vi "1_2_UnifiedCameraCalibration.vi"(5 "um/pix conversion method":T6=1 items=["Strip Centers", "Signal Fit, Left to Right", "Projection + Signal Fit"], 7 "Sharpness assessment method":T5=enum."Mean( Laplacian Convolution )", 8 "error in (no error)":errorcluster, 9 "Strip Pitch (microns)":dbl=74.5 format="%#_13g", 10 "Naming Convention":string="*.png", 11 "Images Directory":path) -> (0 "error out":errorcluster, 3 "Camera calibration results":T3 {"Working distance to stave [mm]" format="%#_13g"})   [LabVIEW 2016]
uses:
  Utils/Controls/All_Enums/Enum_TypeDef_ImageSharpnessAnalysisMethod.ctl
  Utils/Controls/All_Enums/Enum_TypeDef_CameraCalibrationResults.ctl
  Utils/Controls/All_Enums/Ring_TypeDef_PixUmConversionMethod.ctl
  Utils/Controls/All_Enums/Enum_TypeDef_ParabolaFitType.ctl
  <vilib>/Utility/file.llb/Read Delimited Spreadsheet (DBL).vi
panel:
  out "IndexNearOptimal":i32
  out "Array 3":dbl[](array[numeric])
  out "Array 2":dbl[](array[numeric])
  out "Array":dbl[](array[numeric])
  out "Images":T1[](array[plugin-control])
  out "Processing Image #":i32
  in  "Tab Control":T2(tab)
  in  "Name of coordinate file":string="XYZcaptured.csv"
  out "Sharpness vs Height":T4(graph)
  out "Uncertainty on height [mm]":dbl
  out "Optimized height [mm]":dbl
  out "Conversion vs Height":cluster{"all rows":dbl[], dbl[]}[](graph)
  out "Conversion [um/pix]":dbl
  out "Uncertainty on conversion":dbl
  # "CALIBRATE CAMERA Brandeis University - Brookhaven National Laboratory * ATLAS Phase II Inner Tracker Upgrade\nPrimary Authors: H. Herde (hherde@brandeis.edu), C. Nicoloff (cnicolof@wellesley.edu)"
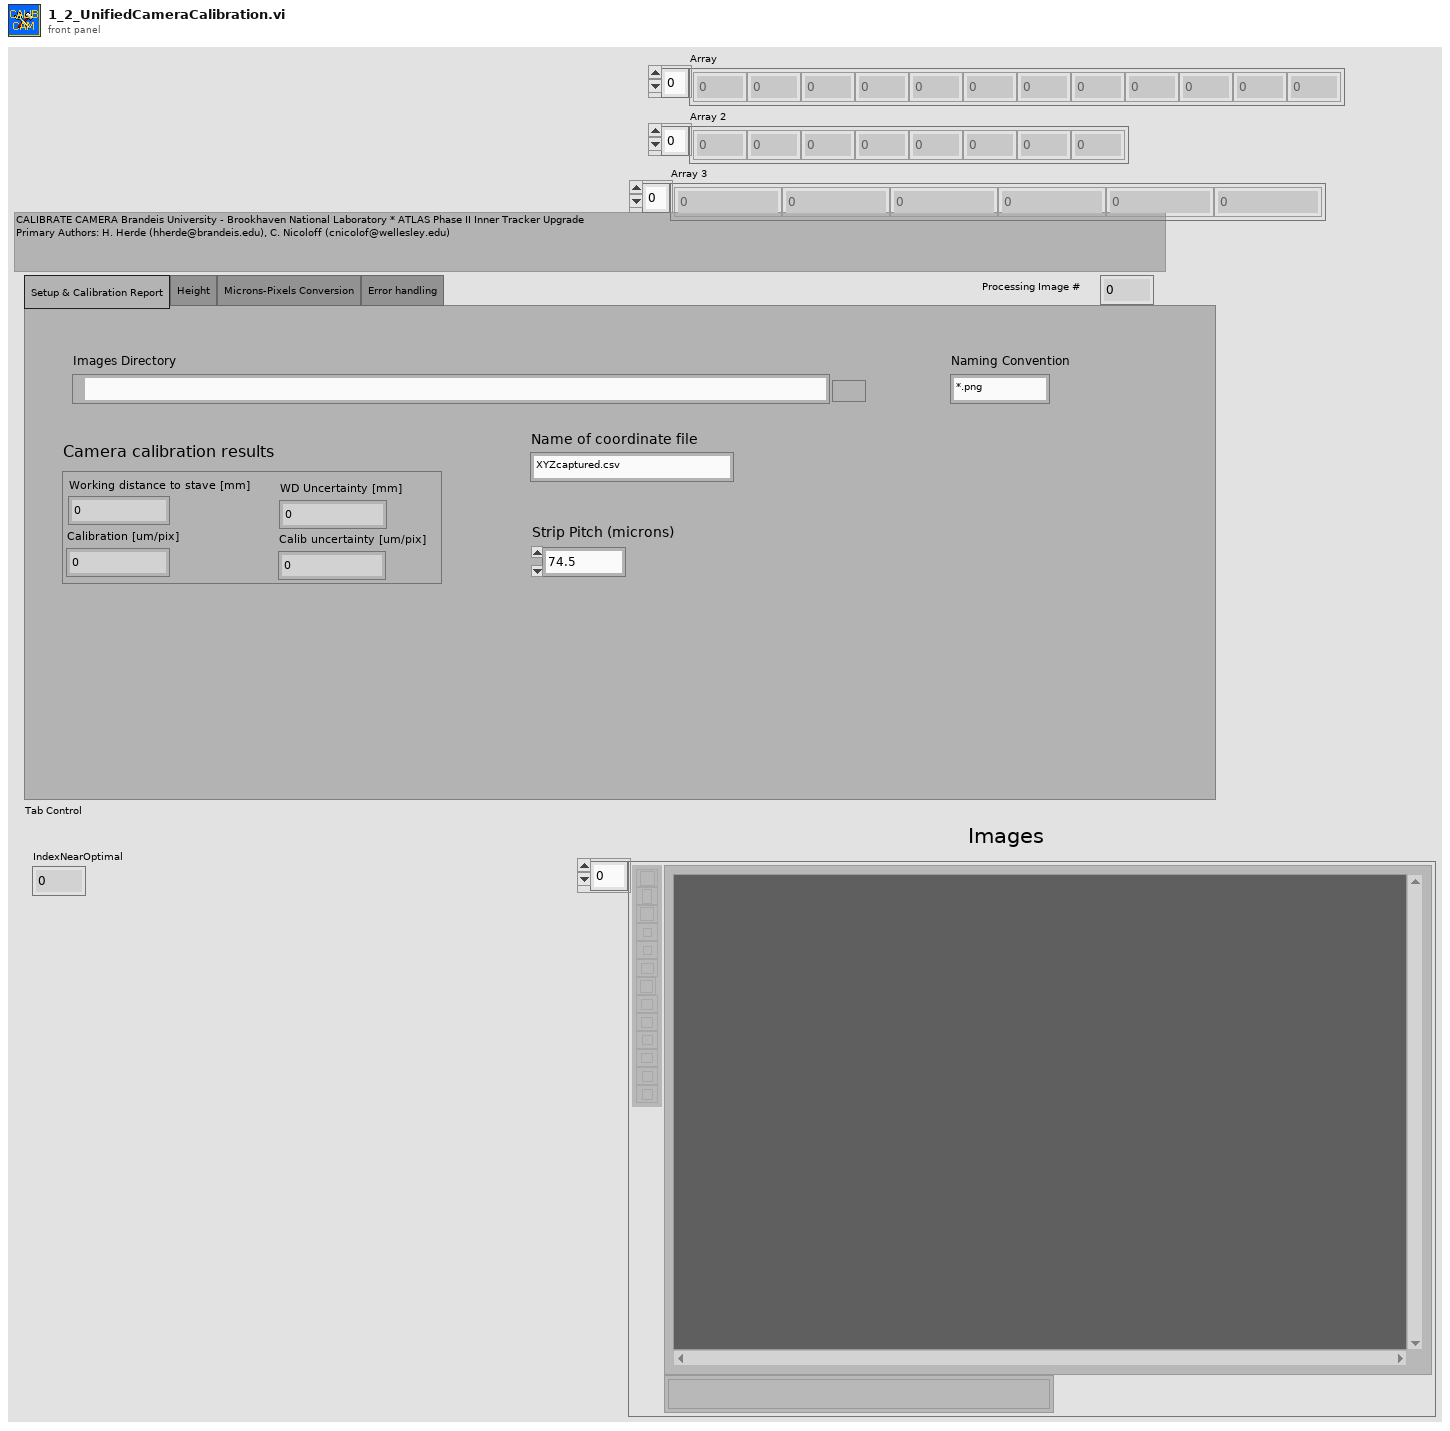
[diagram p1: front panel]
types:
  T1 = typedef "IMAQ Image.ctl" = refnum<image>
  T2 = enum32{"Setup & Calibration Report", "Height", "Microns-Pixels Conversion", "Error handling"}
  T3 = typedef "Enum_TypeDef_CameraCalibrationResults.ctl" = cluster{"Working distance to stave [mm]":dbl, "WD Uncertainty [mm]":dbl, "Calibration [um/pix]":dbl, "Calib uncertainty [um/pix]":dbl}
  T4 = cluster{"Radius bins":dbl[], "Best Gaussian Fit":dbl[]}[]
  T5 = typedef "Enum_TypeDef_ImageSharpnessAnalysisMethod.ctl" = enum16{"sigma( Intensity )", "Mean( Laplacian Convolution )"}
  T6 = typedef "Ring_TypeDef_PixUmConversionMethod.ctl" = u16
  T7 = typedef "Image Type" = u32
  T8 = typedef "Enum_TypeDef_ParabolaFitType.ctl" = enum16{"Expect minimum", "Expect maximum"}
  T9 = typedef "Graph_TypeDef_XY.ctl" = cluster{"Radius bins":dbl[], "Best Gaussian Fit":dbl[]}[]
  T10 = cluster{"Optimized position":dbl, "standard deviation":dbl, "Mean y":dbl, "Uncertainty on mean y":dbl}
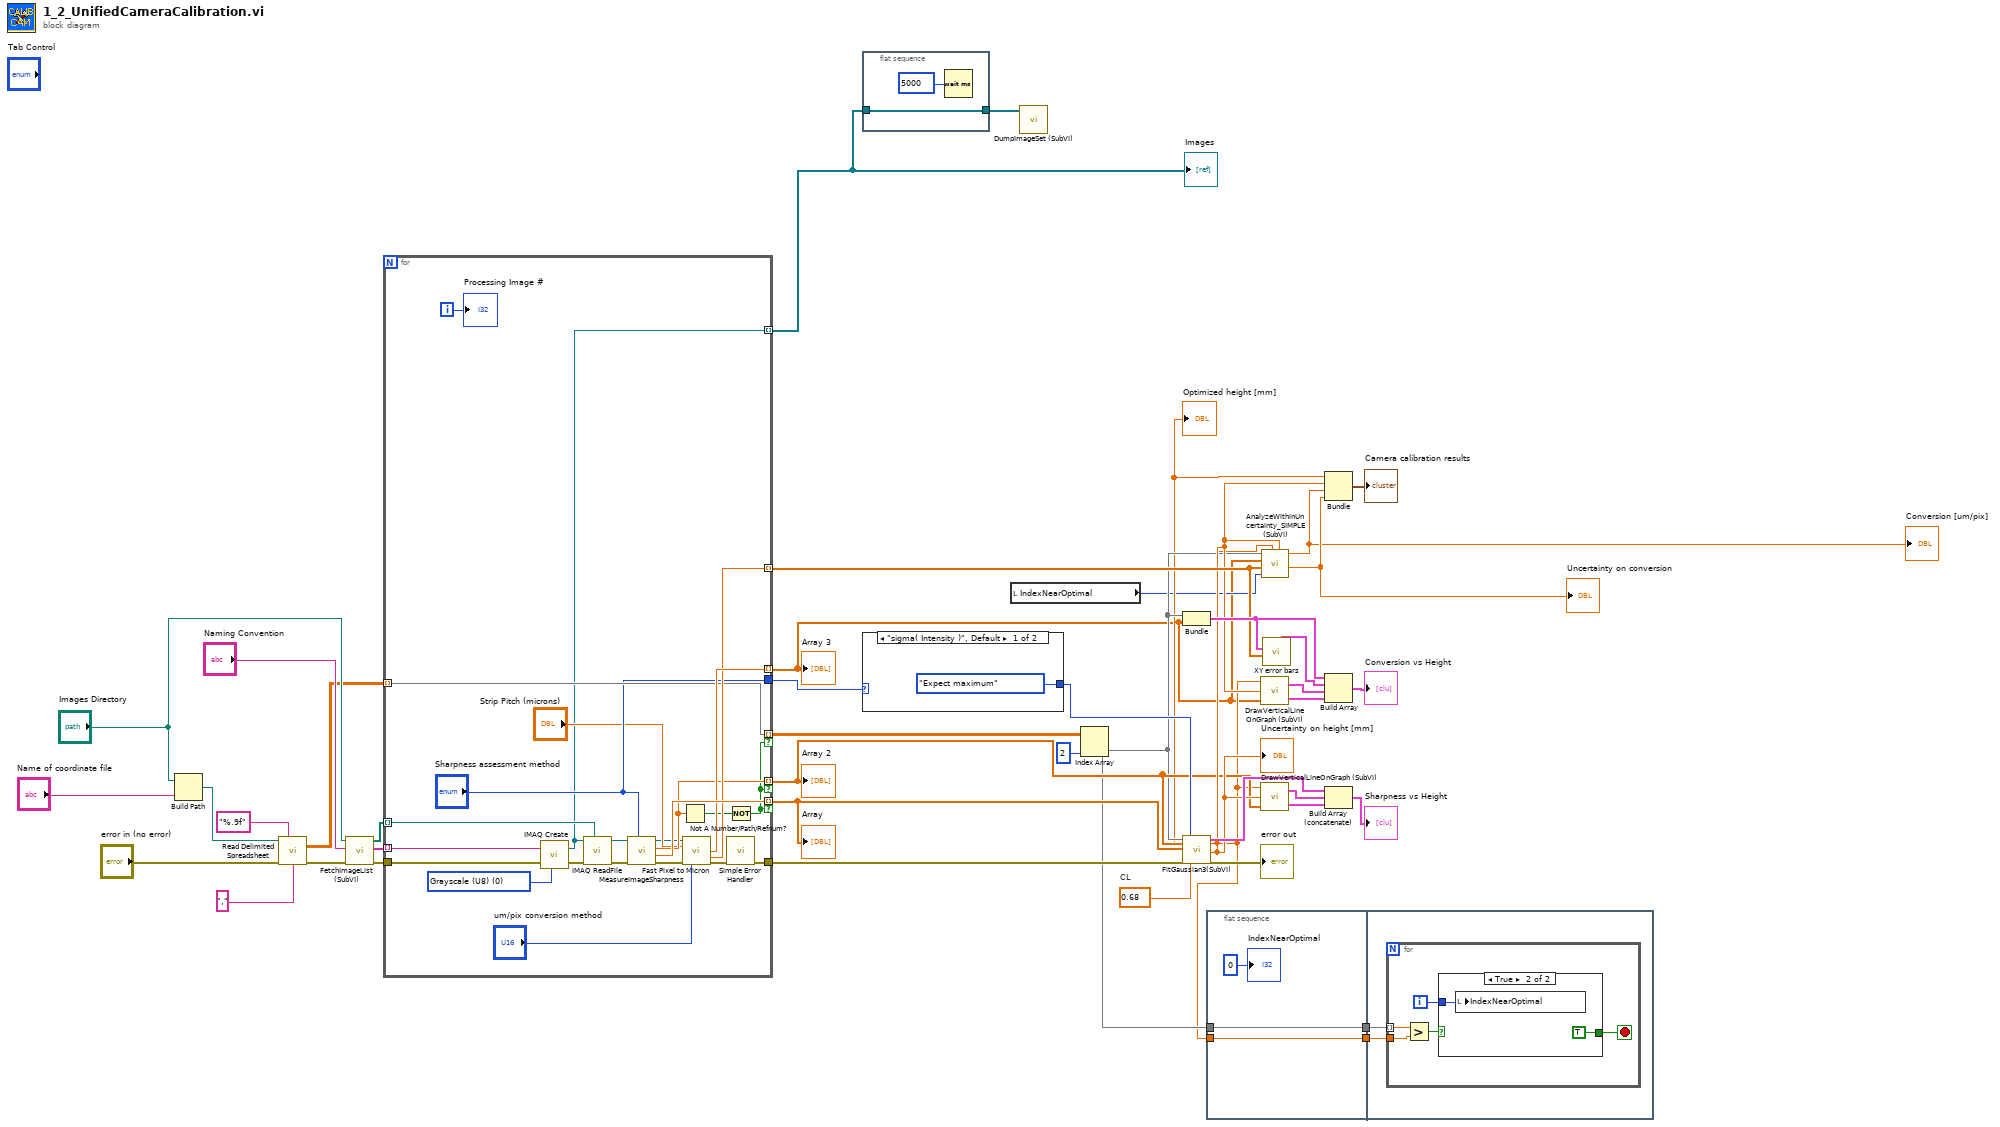
[diagram p0: block diagram]
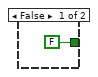
[diagram p2: hidden frame]
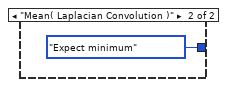
[diagram p3: hidden frame]
diagram:
  w22 = 0.68  # CL
  n1 = Build Path(base path="Images Directory", name or relative path="Name of coordinate file") -> (appended path=w41:path)
  n2 = call-poly <vilib>:"Read Delimited Spreadsheet.vi"("file path (dialog if empty)"=w41, "format (%.3f)"="%.9f", "error in (no error)"="error in (no error)", "delimiter (\\t)"="," ("delimiter (\\t)")) -> ("all rows"=w31:dbl[][], "error out"=w35:errorcluster)  [unwired: 6 in, 4 out]
  n3 = call "FetchImageList (SubVI).vi"("error in (no error)"=w35, "Naming Convention"="Naming Convention", "Images Directory"="Images Directory") -> ("error out"=w42:errorcluster, "List of Image Names"=w32:string[], "List of Image Paths"=w43:path[])  [unwired: 5 in, 1 out]
  n4 = for {
    tunnel: w43 -> [w64] mode=indexing
    tunnel: w32 -> [w66] mode=indexing
    tunnel: w42 -> [w63]
    tunnel: [w54] -> w7 mode=indexing if=w52
    tunnel: [w59] -> w8 mode=indexing if=w52
    tunnel: [w58] -> w1 mode=indexing
    tunnel: [w57] -> w18 mode=indexing
    tunnel: w31 -> [w55] mode=indexing
    tunnel: [w55] -> w30 mode=indexing if=w52
    tunnel: [w49] -> w21
    tunnel: ["Sharpness assessment method"] -> w16
    tunnel: [w44] -> w9 mode=indexing
    i -> [w56]
    w60 = T7 0 items=["Grayscale (U8)", "Grayscale (I16)", "Grayscale (SGL)", "Complex (CSG)", "RGB (U32)", "HSL (U32)", "RGB (U64)", "Grayscale (U16)"] ("Image Type")
    n5 = call "IMAQ Create"("Image Name"=w66, "Image Type"=w60, "error in (no error)"=w63) -> ("New Image"=w44:T1, "error out"=w65:errorcluster)  [unwired: 2 in]
    n6 = call "IMAQ ReadFile"("File Path"=w64, "error in (no error)"=w65, "Image"=w44) -> ("error out"=w62:errorcluster, "Image Out"=w48:T1)  [unwired: 4 in, 3 out]
    n7 = call "MeasureImageSharpness.vi"("Method"="Sharpness assessment method", "error in (no error)"=w62, "Image In"=w48) -> ("error out"=w61:errorcluster, "Sharpness Uncertainty"=w59:dbl, "Sharpness"=w54:dbl, "Image Out"=w45:T1)  [unwired: 5 in]
    n8 = Not A Number/Path/Refnum?(number/path/refnum=w54) -> (NaN/Path/Refnum?=w53:bool)
    n9 = call "Fast Pixel to Micron.vi"("Refnum In"=w45, "Strip Pitch (microns)"="Strip Pitch (microns)", "error in (no error)"=w61, "Conversion Method"="um/pix conversion method") -> ("Microns/Pixel (Corrected)"=w58:dbl, "Error (Corrected)"=w57:dbl, "error out"=w50:errorcluster)  [unwired: 5 in, 4 out]
    n10 = call <vilib>:"Simple Error Handler.vi"("error in (no error)"=w50) -> ("error out"=w49:errorcluster)  [unwired: 4 in, 4 out]
    n11 = Not(x=w53) -> (.not. x?=w52:bool)
    "Processing Image #" <- w56
  }
  "Images" <- w9
  "Array" <- w8
  "Array 2" <- w7
  "Array 3" <- w1
  n12 = flat-sequence {
    tunnel: [w67] -> w10
    tunnel: w9 -> [w67]
    frame #0 {
      n13 = Wait (ms)(milliseconds to wait=u32 5000) -> ()  [unwired: 1 out]
    }
  }
  n14 = case shown="\"sigma( Intensity )\", Default" w16 {
    tunnel: [Enum_TypeDef_ParabolaFitType."Expect maximum" ("Fit type") Enum_TypeDef_ParabolaFitType."Expect minimum" ("Fit type")] -> w15
    frame "sigma( Intensity )", Default {
    }
    frame "Mean( Laplacian Convolution )" {
    }
  }
  n15 = local read "IndexNearOptimal"() -> (w2:i32)
  n16 = call "DumpImageSet (SubVI).vi"("Calibrated Image Array"=w10) -> ()  [unwired: 7 in, 1 out]
  n17 = Index Array(array=w30, index (col)=2 ("disabled index (col)")) -> (element=w6:dbl[])  [unwired: 1 in]
  n18 = Bundle("all rows"=w6, w1) -> (w20:cluster{"all rows":dbl[], dbl[]})  [unwired: 1 in]
  n19 = call "FitGaussian3(SubVI).vi"("x values"=w6, "y values"=w7, "delta y values"=w8, "error in"=w21, "Fit type"=w15, "confidence level"=w22) -> ("Plot"=w29:T9, "Optimized position"=w5:dbl, "standard deviation"=w12:dbl, "error out"=→"error out":errorcluster)  [unwired: 8 in, 2 out]
  "Uncertainty on height [mm]" <- w12
  "Optimized height [mm]" <- w5
  n20 = flat-sequence {
    tunnel: w5 -> [w72]
    tunnel: w6 -> [w73]
    tunnel: [w73] -> w4
    tunnel: [w72] -> w3
    tunnel: w4 -> [w75]
    tunnel: w3 -> [w74]
    frame #0 {
      "IndexNearOptimal" <- 0
    }
    frame #1 {
      n21 = for {
        tunnel: w75 -> [w80] mode=indexing
        tunnel: w74 -> [w79]
        i -> [w77]
        stop <- w76 stop-if-true
        n22 = Greater?(x=w80, y=w79) -> (0:w78:bool)
        n23 = case shown="True" w78 {
          tunnel: w77 -> [_ w83]
          tunnel: [FALSE TRUE] -> w76
          frame False {
          }
          frame True {
            n24 = local write "IndexNearOptimal"(w83) -> ()
          }
        }
      }
    }
  }
  n25 = call "DrawVerticalLineOnGraph (SubVI).vi"("Array"=w1, "value uncertainty"=w12, "x = value"=w5) -> ("X error bars"=w26:cluster{dbl[], dbl[]}, "Line at x = value"=w27:cluster{dbl[], dbl[]})
  n26 = call "DrawVerticalLineOnGraph (SubVI).vi"("Array"=w7, "value uncertainty"=w12, "x = value"=w5) -> ("X error bars"=w24:cluster{dbl[], dbl[]}, "Line at x = value"=w25:cluster{dbl[], dbl[]})
  n27 = call "AnalyzeWithinUncertainty_SIMPLE (SubVI).vi"("Uncertainty on mean x"=w12, "Mean x"=w5, "Numeric"=w2, "y uncertainties"=w18, "y values"=w1, "x values"=w6) -> ("Uncertainty on mean y"=w13:dbl, "Mean y"=w11:dbl)  [unwired: 3 in, 1 out]
  "Conversion [um/pix]" <- w11
  "Uncertainty on conversion" <- w13
  n28 = call "XY error bars.vi"("XY plot"=w20, "Xerror"=w18) -> ("Y error bars"=w19:cluster{dbl[], dbl[]})  [unwired: 6 in, 2 out]
  n29 = Bundle("Optimized position"=w5, "standard deviation"=w12, "Mean y"=w11, "Uncertainty on mean y"=w13) -> (→"Camera calibration results":T10)  [unwired: 1 in]
  n30 = Build Array(w20, w19, w27, w26) -> (→"Conversion vs Height":cluster{"all rows":dbl[], dbl[]}[])
  n31 = Build Array (concatenate)(w29, w25, w24) -> (→"Sharpness vs Height":T9)
